vi "GradientSearchGraph.vi"(0 "System no.":i32=1 min=1 step=1, 2 "X Axis":u16(ring) items=["1", "2", "3", "4", "5", "6", "7", "8", "9", "10", "11", "12"], 3 "Y Axis":u16(ring) items=["1", "2", "3", "4", "5", "6", "7", "8", "9", "10", "11", "12"]) -> ()   [LabVIEW 2020]
doc: "This VI shows the position of the axes that are used for the selected gradient search routines.\nIf Raw Data? is selected, the current position (POS?) is shown instead of using the gradient search center and radius.\nThis VI can also be used to visualize the position even if no scan is running."
uses:
  Message Cluster.ctl
  C:/ProgramData/PI/LabVIEW/Low Level/GeneralCommands/Global2 (Array).vi
panel:
  in  "OverrideClone":bool
  out "Y Position":dbl
  out "X Position":dbl
  in  "Scan Index":i32
  in  "GS Name":string
  in  "Raw Data":bool
  out "XY Graph":cluster{dbl[], dbl[]}(graph)
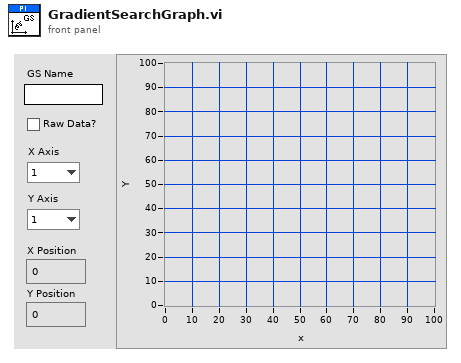
[diagram p1: front panel]
types:
  T1 = typedef "Message Cluster.ctl" = cluster{"Message":string, "Message Data":variant}
  T2 = cluster{"Gradient Scan Names":string[], "Dither Radius":dbl[], "Scan axis center":dbl[], "Step axis center":dbl[]}
  T3 = typedef "Controller names.ctl" = enum16{"None", "Analog", "C-702", "C-413", "C-414", "C-843", "C-843.PM", "C-844", "C-848", "C-865", "C-866", "C-867", "C-877", "C-880", "C-884", "C-885", "C-886", "C-887", "C-891", "E-135", "E-516", "E-517", "E-518", "E-709", "E-710", "E-712", "E-725", "E-727", "E-753", "E-754", "E-755", "E-761", "E-816", "E-861", "E-870", "E-871", "E-872", "E-873", "E-874", "F-206", "HydraPollux", "M-840", "M-850", "M-8X0", "Mercury", "Mercury_GCS", "PI_GCS2"}
  T4 = cluster{"Conn. axes":string[], "Controller name":T3}[]
  T5 = cluster{"Conn. axes":string[], "Controller name":T3}
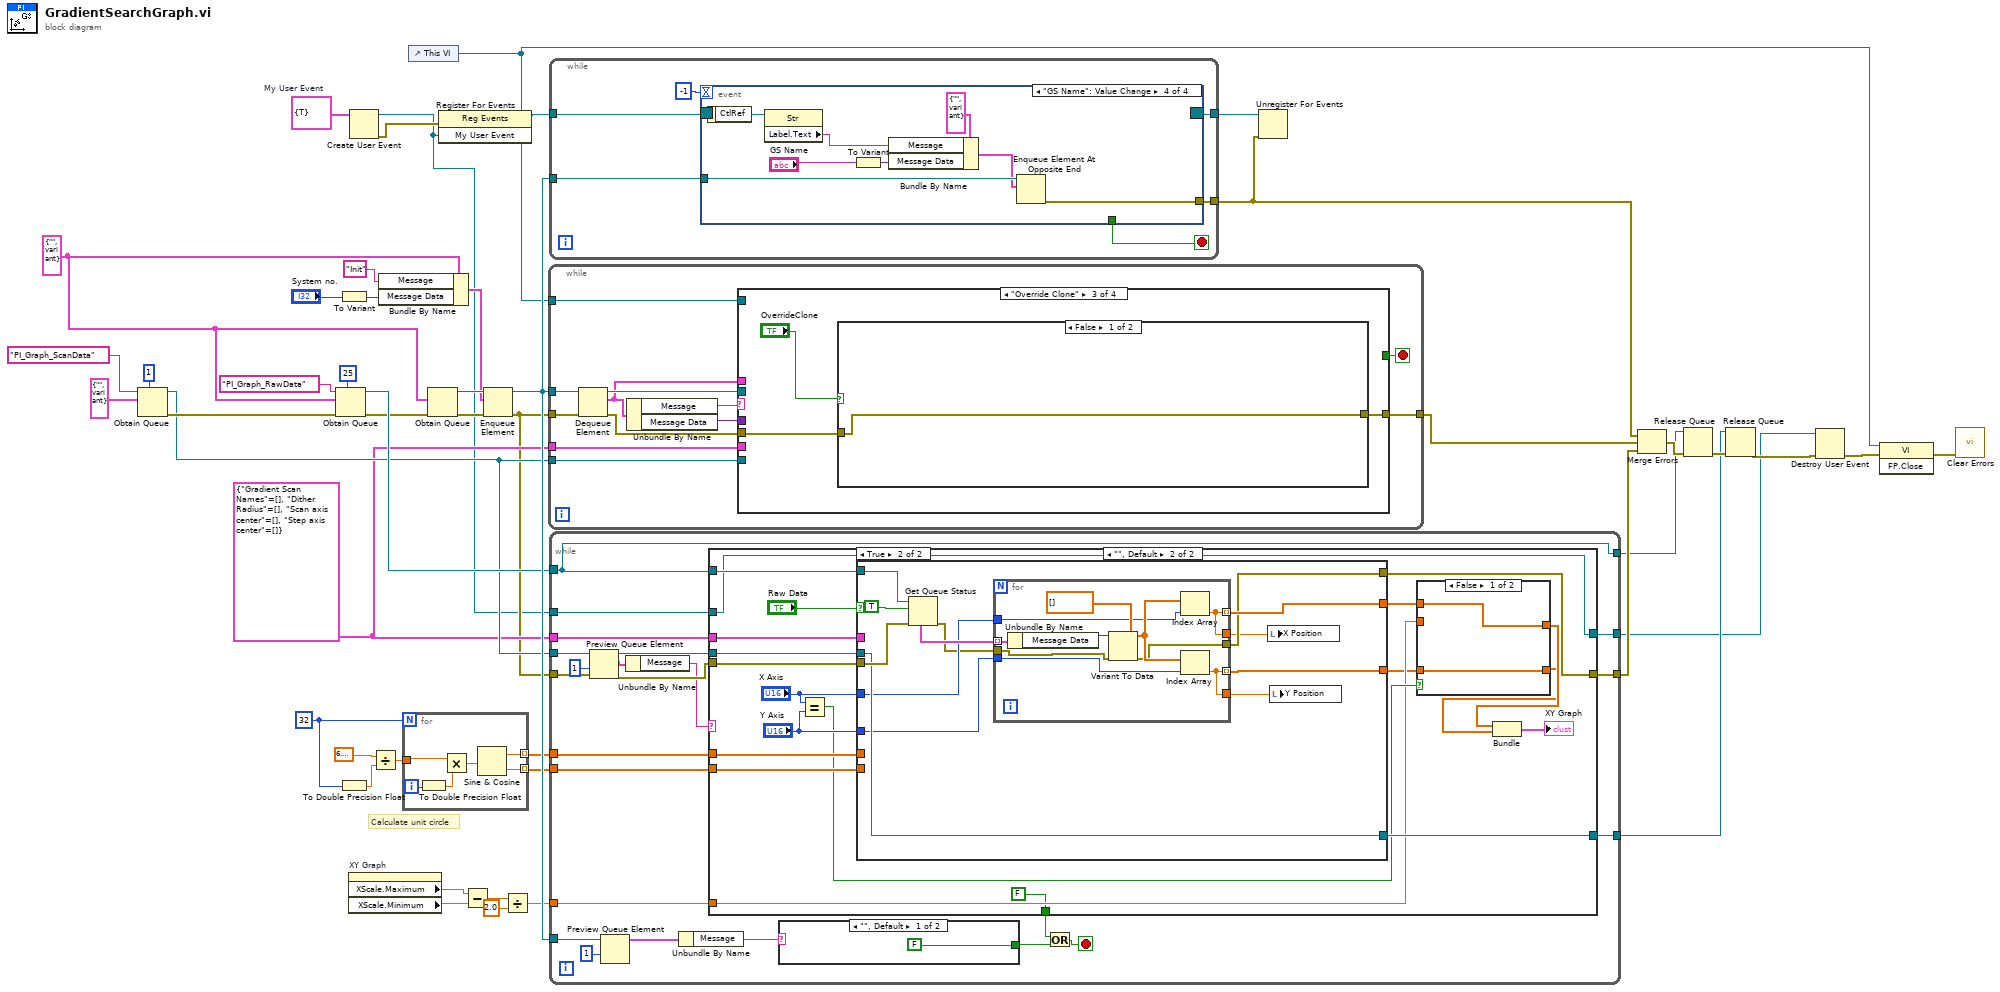
[diagram p0: block diagram]
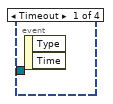
[diagram p2: hidden frame]
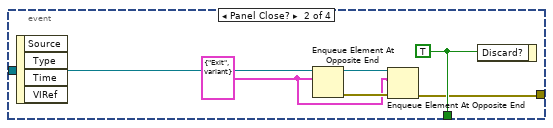
[diagram p3: hidden frame]
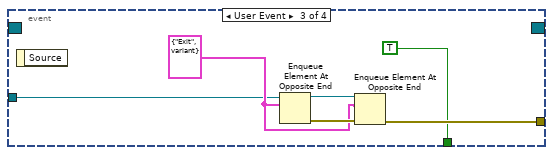
[diagram p4: hidden frame]
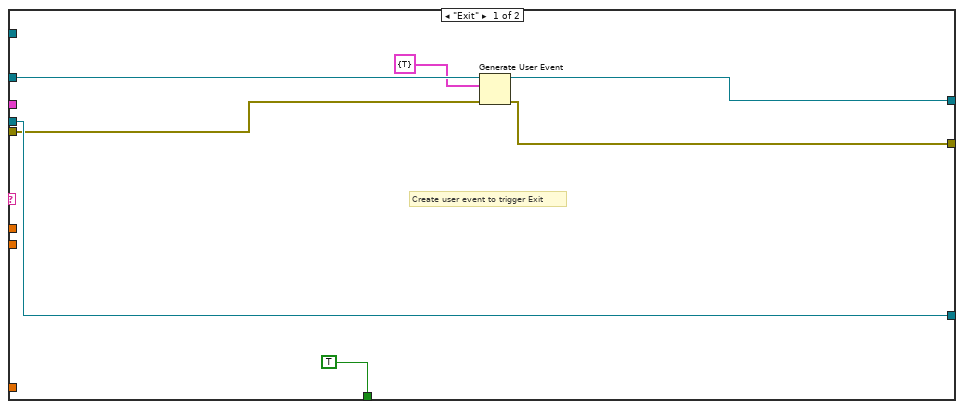
[diagram p5: hidden frame]
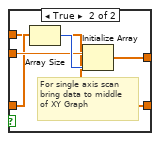
[diagram p6: hidden frame]
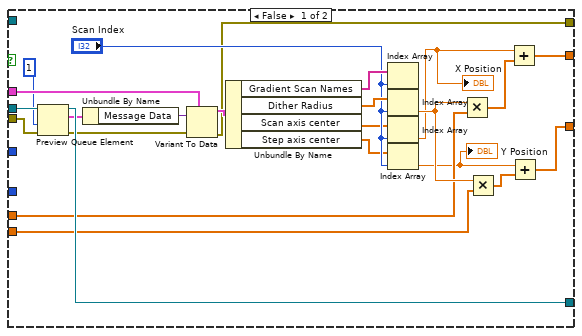
[diagram p7: hidden frame]
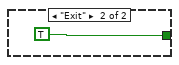
[diagram p8: hidden frame]
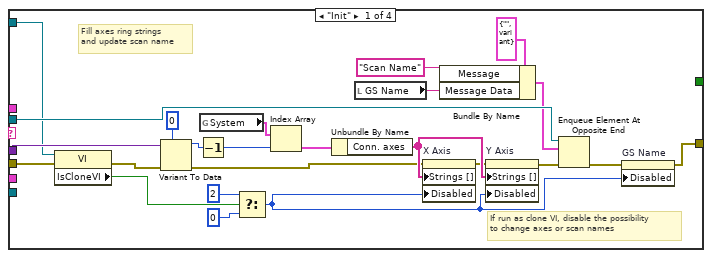
[diagram p9: hidden frame]
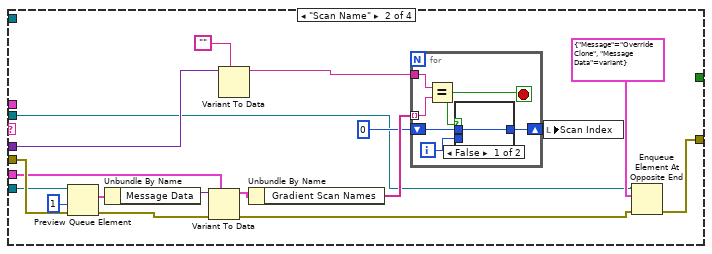
[diagram p10: hidden frame]
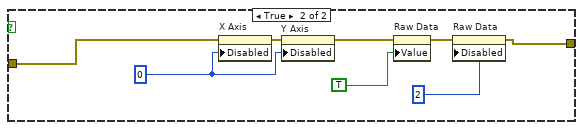
[diagram p12: hidden frame]
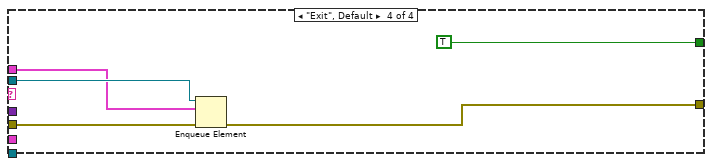
[diagram p13: hidden frame]
diagram:
  w2 = cluster{"Trigger":bool} {"Trigger"=TRUE}  # My User Event
  w22 = T2 {"Gradient Scan Names"=[], "Dither Radius"=[], "Scan axis center"=[], "Step axis center"=[]} ("cluster")
  w30 = 32
  w13 = T1 {"Message"="", "Message Data"=variant} ("Message Cluster")
  # "Calculate unit circle"
  n1 = Obtain Queue(max queue size (-1, unlimited)=1, name (unnamed)="PI_Graph_ScanData", element data type=T1 {"Message"="", "Message Data"=variant} ("Message Cluster")) -> (queue out=w23:refnum<queue>, error out=w26:errorcluster)  [unwired: 2 in, 1 out]
  n2 = Obtain Queue(max queue size (-1, unlimited)=25, name (unnamed)="PI_Graph_RawData", element data type=w13, error in (no error)=w26) -> (queue out=w40:refnum<queue>, error out=w39:errorcluster)  [unwired: 1 in, 1 out]
  n3 = To Variant(anything="System no.") -> (Variant=w42:variant)
  n4 = To Double Precision Float(number=w30) -> (double precision float=w31:dbl)
  n5 = property on="XY Graph" class="XYGraph (strict)"() -> ("XScale.Maximum"=w18:dbl, "XScale.Minimum"=w17:dbl)  [unwired: 2 in, 2 out]
  n6 = Create User Event(user event datatype=w2) -> (user event=w8:refnum<user-event>, error out=w9:errorcluster)  [unwired: 1 in]
  n7 = Divide(x=6.283185307179586, y=w31) -> (x/y=w29:dbl)
  n8 = Bundle By Name(cluster=w13, "Message"="Init", "Message Data"=w42) -> (w44:T1)
  n9 = for {
    N: w30 -> [_]
    tunnel: w29 -> [w53]
    tunnel: [w49] -> w16 mode=indexing
    tunnel: [w48] -> w21 mode=indexing
    i -> [w52]
    n10 = To Double Precision Float(number=w52) -> (double precision float=w51:dbl)
    n11 = Multiply(x=w53, y=w51) -> (x*y=w50:dbl)
    n12 = Sine & Cosine(0:w50) -> (1:w49:dbl, 2:w48:dbl)
  }
  n13 = control-ref of="This VI"() -> (w11:refnum<vi>)
  n14 = Obtain Queue(element data type=w13, error in (no error)=w39) -> (queue out=w45:refnum<queue>, error out=w46:errorcluster)  [unwired: 2 in, 2 out]
  n15 = register-events(error in=w9, w8) -> (reference out=w10:refnum<event-registration>)  [unwired: 1 in, 1 out]
  n16 = Subtract(x=w18, y=w17) -> (x-y=w19:dbl)
  n17 = Enqueue Element(queue=w45, element=w44, error in (no error)=w46) -> (queue out=w47:refnum<queue>, error out=w14:errorcluster)  [unwired: 2 out]
  n18 = Divide(x=w19, y=2.0) -> (x/y=w15:dbl)
  n19 = while {
    tunnel: w47 -> [w62]
    tunnel: w23 -> [w56]
    tunnel: w22 -> [w55]
    tunnel: w11 -> [w54]
    tunnel: w14 -> [w63]
    tunnel: [w64] -> w36
    stop <- w65 stop-if-true
    n20 = Dequeue Element(queue=w62, error in (no error)=w63) -> (queue out=w61:refnum<queue>, element=w57:T1, error out=w60:errorcluster)  [unwired: 2 out]
    n21 = Unbundle By Name(w57) -> ("Message"=w59:string, "Message Data"=w58:variant)
    n22 = case "Message Cases" shown="\"Override Clone\"" w59 {
      tunnel: w61 -> [w80 w90 _ w129]
      tunnel: w60 -> [w75 w107 w117 w131]
      tunnel: [w70 w92 w116 w130] -> w64
      tunnel: [_ _ _ TRUE] -> w65
      tunnel: w58 -> [w88 w105 _ _]
      tunnel: w57 -> [_ _ _ w128]
      tunnel: w56 -> [_ w91 _ _]
      tunnel: w55 -> [_ w95 _ _]
      tunnel: w54 -> [w73 _ _ _]
      frame "Init" {
        # "If run as clone VI, disable the possibility\nto change axes or scan names"
        # "Fill axes ring strings\nand update scan name"
        n23 = property class="VI"(reference=w73, error in=w75) -> (error out=w74:errorcluster, "IsCloneVI"=w69:bool)  [unwired: 1 out]
        n24 = Variant To Data(error in=w74, type=0, Variant=w88) -> (data=w83:i32, error out=w72:errorcluster)
        n25 = Decrement(x=w83) -> (x-1=w82:i32)
        n26 = global read "Global2 (Array).vi" "System"() -> (w87:T4)
        n27 = Select(t=u8 2 ("Disabled"), s=w69, f=u8 0 ("Disabled")) -> (s? t:f=w68:u8)
        n28 = Index Array(array=w87, index=w82) -> (element=w86:T5)
        n29 = Unbundle By Name(w86) -> ("Conn. axes"=w85:string[])
        n30 = local read "GS Name"() -> (w78:string)
        n31 = property on="X Axis" class="Ring (strict)"(error in=w72, "Strings []"=w85, "Disabled"=w68) -> (error out=w84:errorcluster)  [unwired: 1 in, 1 out]
        n32 = Bundle By Name(cluster=T1 {"Message"="", "Message Data"=variant} ("element"), "Message"="Scan Name", "Message Data"=w78) -> (w77:T1)
        n33 = property on="Y Axis" class="Ring (strict)"(error in=w84, "Strings []"=w85, "Disabled"=w68) -> (error out=w81:errorcluster)  [unwired: 1 in, 1 out]
        n34 = Enqueue Element At Opposite End(queue=w80, element=w77, error in (no error)=w81) -> (error out=w71:errorcluster)  [unwired: 3 out]
        n35 = property on="GS Name" class="Str"(error in=w71, "Disabled"=w68) -> (error out=w70:errorcluster)  [unwired: 1 in, 1 out]
      }
      frame "Scan Name" {
        n36 = Preview Queue Element(queue=w91, timeout in ms (-1)=1, error in (no error)=w107) -> (element=w103:T1, error out=w101:errorcluster)  [unwired: 2 out]
        n37 = Unbundle By Name(w103) -> ("Message Data"=w102:variant)
        n38 = Variant To Data(error in=w101, type=w95, Variant=w102) -> (data=w100:T2, error out=w93:errorcluster)
        n39 = Variant To Data(type="", Variant=w105) -> (data=w98:string)  [unwired: 1 in, 1 out]
        n40 = Unbundle By Name(w100) -> ("Gradient Scan Names"=w99:string[])
        n41 = for {
          tunnel: w99 -> [w113] mode=indexing
          tunnel: w98 -> [w112]
          shift-right: [w109] -> w97
          shift-left: 0 -> [w108]
          i -> [w111]
          stop <- w110 stop-if-true
          n42 = Equal?(x=w112, y=w113) -> (x = y?=w110:bool)
          n43 = case shown="False" w110 {
            tunnel: w111 -> [_ w115]
            tunnel: [w114 w115] -> w109
            tunnel: w108 -> [w114 _]
            frame False {
            }
            frame True {
            }
          }
        }
        n44 = local write "Scan Index"(w97) -> ()
        n45 = Enqueue Element At Opposite End(queue=w90, element=T1 {"Message"="Override Clone", "Message Data"=variant}, error in (no error)=w93) -> (error out=w92:errorcluster)  [unwired: 3 out]
      }
      frame "Override Clone" {
        n46 = case shown="False" "OverrideClone" {
          tunnel: w117 -> [w119 w125]
          tunnel: [w119 w120] -> w116
          frame False {
          }
          frame True {
            w126 = 0
            n47 = property on="X Axis" class="Ring (strict)"(error in=w125, "Disabled"=w126) -> (error out=w127:errorcluster)  [unwired: 1 in, 1 out]
            n48 = property on="Y Axis" class="Ring (strict)"(error in=w127, "Disabled"=w126) -> (error out=w124:errorcluster)  [unwired: 1 in, 1 out]
            n49 = property on="Raw Data" class="Bool (strict)"(error in=w124, "Value"=TRUE) -> (error out=w122:errorcluster)  [unwired: 1 in, 1 out]
            n50 = property on="Raw Data" class="Bool (strict)"(error in=w122, "Disabled"=u8 2) -> (error out=w120:errorcluster)  [unwired: 1 in, 1 out]
          }
        }
      }
      frame "Exit", Default {
        n51 = Enqueue Element(queue=w129, element=w128, error in (no error)=w131) -> (error out=w130:errorcluster)  [unwired: 3 out]
      }
    }
  }
  n52 = while {
    tunnel: w47 -> [w137]
    tunnel: [w136] -> w6
    tunnel: w10 -> [w134]
    tunnel: [w133] -> w7
    stop <- w138 stop-if-true
    n53 = event shown="[3] \"GS Name\": Value Change" {
      selector: w134 -> [_ _ _ _]
      dyn-events: [_ _ _ _] -> w133
      timeout: -1 -> [_ _ _ _]
      tunnel: [_ w144 TRUE _] -> w138
      tunnel: w137 -> [_ w143 w145 w157]
      tunnel: [_ w139 w147 w158] -> w136
      event Timeout {
        n54 = event-data() -> ()  [unwired: 3 out]
      }
      event Panel Close? {
        w140 = T1 {"Message"="Exit", "Message Data"=variant} ("element")
        w144 = TRUE
        n55 = event-data() -> ()  [unwired: 5 out]
        n56 = Enqueue Element At Opposite End(queue=w143, element=w140) -> (queue out=w141:refnum<queue>, error out=w142:errorcluster)  [unwired: 1 in, 2 out]
        n57 = Enqueue Element At Opposite End(queue=w141, element=w140, error in (no error)=w142) -> (error out=w139:errorcluster)  [unwired: 3 out]
        n58 = event-data("Discard?"=w144) -> ()  [unwired: 1 in, 1 out]
      }
      event User Event {
        w148 = T1 {"Message"="Exit", "Message Data"=variant} ("element")
        n59 = event-data() -> ()  [unwired: 2 out]
        n60 = Enqueue Element At Opposite End(queue=w145, element=w148) -> (queue out=w149:refnum<queue>, error out=w150:errorcluster)  [unwired: 1 in, 2 out]
        n61 = Enqueue Element At Opposite End(queue=w149, element=w148, error in (no error)=w150) -> (error out=w147:errorcluster)  [unwired: 3 out]
      }
      event "GS Name": Value Change {
        n62 = event-data() -> ("CtlRef"=w152:refnum<vi>)  [unwired: 1 out]
        n63 = property class="Str"(reference=w152) -> ("Label.Text"=w151:string)  [unwired: 1 in, 2 out]
        n64 = To Variant(anything="GS Name") -> (Variant=w153:variant)
        n65 = Bundle By Name(cluster=T1 {"Message"="", "Message Data"=variant} ("Message Cluster"), "Message"=w151, "Message Data"=w153) -> (w155:T1)
        n66 = Enqueue Element At Opposite End(queue=w157, element=w155) -> (error out=w158:errorcluster)  [unwired: 1 in, 3 out]
      }
    }
  }
  n67 = while {
    tunnel: w40 -> [w177]
    tunnel: w47 -> [w165]
    tunnel: [w177] -> w33
    tunnel: w23 -> [w171]
    tunnel: [w176] -> w24
    tunnel: w22 -> [w175]
    tunnel: w16 -> [w174]
    tunnel: w21 -> [w173]
    tunnel: w15 -> [w172]
    tunnel: w8 -> [w160]
    tunnel: [w159] -> w3
    tunnel: w14 -> [w169]
    tunnel: [w178] -> w35
    stop <- w161 stop-if-true
    n68 = Preview Queue Element(queue=w171, timeout in ms (-1)=1, error in (no error)=w169) -> (queue out=w170:refnum<queue>, element=w167:T1, error out=w168:errorcluster)  [unwired: 1 out]
    n69 = Preview Queue Element(queue=w165, timeout in ms (-1)=1) -> (element=w181:T1)  [unwired: 1 in, 3 out]
    n70 = Unbundle By Name(w167) -> ("Message"=w166:string)
    n71 = Unbundle By Name(w181) -> ("Message"=w180:string)
    n72 = case shown="\"\", Default" w166 {
      tunnel: [w183 w207] -> w178
      tunnel: w177 -> [_ w206]
      tunnel: [w188 w204] -> w176
      tunnel: w175 -> [_ w203]
      tunnel: w174 -> [_ w202]
      tunnel: w173 -> [_ w201]
      tunnel: w172 -> [_ w197]
      tunnel: w170 -> [w188 w193]
      tunnel: w168 -> [w184 w192]
      tunnel: [TRUE FALSE] -> w162
      tunnel: w160 -> [w186 w190]
      tunnel: [w185 w190] -> w159
      frame "Exit" {
        # "Create user event to trigger Exit"
        n73 = Generate User Event(user event=w186, event data cluster=cluster{bool} {TRUE} ("event data"), error in=w184) -> (user event out=w185:refnum<user-event>, error out=w183:errorcluster)  [unwired: 1 in]
      }
      frame "", Default {
        n74 = Equal?(x="X Axis", y="Y Axis") -> (x = y?=w198:bool)
        n75 = case shown="True" "Raw Data" {
          tunnel: [w220 w252] -> w195
          tunnel: w192 -> [w237 w250]
          tunnel: [w224 w242] -> w207
          tunnel: w206 -> [_ w248]
          tunnel: [w221 w244] -> w189
          tunnel: w193 -> [w239 w247]
          tunnel: [w238 w247] -> w204
          tunnel: w203 -> [w234 _]
          tunnel: w202 -> [w219 _]
          tunnel: w201 -> [w218 _]
          tunnel: "X Axis" -> [_ w246]
          tunnel: "Y Axis" -> [_ w245]
          frame False {
            n76 = Preview Queue Element(queue=w239, timeout in ms (-1)=1, error in (no error)=w237) -> (queue out=w238:refnum<queue>, element=w236:T1, error out=w223:errorcluster)  [unwired: 1 out]
            n77 = Unbundle By Name(w236) -> ("Message Data"=w235:variant)
            n78 = Variant To Data(error in=w223, type=w234, Variant=w235) -> (data=w233:T2, error out=w224:errorcluster)
            n79 = Unbundle By Name(w233) -> ("Gradient Scan Names"=w232:string[], "Dither Radius"=w231:dbl[], "Scan axis center"=w229:dbl[], "Step axis center"=w228:dbl[])
            n80 = Index Array(array=w232, index="Scan Index") -> ()  [unwired: 1 out]
            n81 = Index Array(array=w231, index="Scan Index") -> (element=w227:dbl)
            n82 = Index Array(array=w229, index="Scan Index") -> (element=w222:dbl)
            "X Position" <- w222
            n83 = Index Array(array=w228, index="Scan Index") -> (element=w216:dbl)
            "Y Position" <- w216
            n84 = Multiply(x=w227, y=w219) -> (x*y=w225:dbl[])
            n85 = Multiply(x=w227, y=w218) -> (x*y=w226:dbl[])
            n86 = Add(x=w222, y=w225) -> (x+y=w221:dbl[])
            n87 = Add(x=w216, y=w226) -> (x+y=w220:dbl[])
          }
          frame True {
            n88 = Get Queue Status(queue=w248, return elements? (F)=TRUE, error in (no error)=w250) -> (error out=w243:errorcluster, elements=w251:T1[])  [unwired: 6 out]
            n89 = for {
              tunnel: w251 -> [w262] mode=indexing
              tunnel: [w253] -> w252 mode=indexing
              tunnel: [w254] -> w244 mode=indexing
              tunnel: w246 -> [w258]
              tunnel: w245 -> [w257]
              tunnel: w243 -> [w256]
              tunnel: [w255] -> w242
              tunnel: [w254] -> w241
              tunnel: [w253] -> w240
              n90 = Unbundle By Name(w262) -> ("Message Data"=w260:variant)
              n91 = Variant To Data(error in=w256, type=dbl[] [] ("Position"), Variant=w260) -> (data=w261:dbl[], error out=w255:errorcluster)
              n92 = Index Array(array=w261, index=w258) -> (element=w254:dbl)
              n93 = Index Array(array=w261, index=w257) -> (element=w253:dbl)
            }
            n94 = local write "X Position"(w241) -> ()
            n95 = local write "Y Position"(w240) -> ()
          }
        }
        n96 = case shown="False" w198 {
          tunnel: w189 -> [w210 w211]
          tunnel: [w210 w214] -> w196
          tunnel: w197 -> [_ w213]
          tunnel: w195 -> [w209 w212]
          tunnel: [w209 w211] -> w194
          frame False {
          }
          frame True {
            # "For single axis scan\nbring data to middle\nof XY Graph"
            n97 = Array Size(array=w212) -> (size(s)=w215:i32)
            n98 = Initialize Array(w213, w215) -> (w214:dbl[])
          }
        }
        n99 = Bundle(w196, w194) -> (→"XY Graph":cluster{dbl[], dbl[]})  [unwired: 1 out]
      }
    }
    n100 = case shown="\"\", Default" w180 {
      tunnel: [FALSE TRUE] -> w163
      frame "", Default {
      }
      frame "Exit" {
      }
    }
    n101 = Or(x=w162, y=w163) -> (x .or. y?=w161:bool)
  }
  n102 = Unregister For Events(event registration refnum=w7, error in=w6) -> ()  [unwired: 1 out]
  n103 = Merge Errors(w6, w36, w35) -> (w34:errorcluster)
  n104 = Release Queue(queue=w33, error in (no error)=w34) -> (error out=w25:errorcluster)  [unwired: 3 out]
  n105 = Release Queue(queue=w24, error in (no error)=w25) -> (error out=w5:errorcluster)  [unwired: 3 out]
  n106 = Destroy User Event(user event=w3, error in=w5) -> (error out=w4:errorcluster)
  n107 = invoke class="VI" method="FP.Close"(reference=w11, error in=w4) -> (error out=w1:errorcluster)  [unwired: 1 in, 2 out]
  n108 = call <vilib>:"Clear Errors.vi"("error in (no error)"=w1) -> ()  [unwired: 1 in, 6 out]
